vi "ITC503 -- scan ITC LTC state.vi"(6 "error logfile path":path, 7 "disable interaction with itc":T1(ring)=enum."do not use oxford ITC", 8 "error in":errorcluster, 11 "state IN":T3={"LTC21 Address"="GPIB0::15::INSTR", "ITC503 Address"="GPIB0::24::INSTR", "ITC temperature"=138.96, "ITC set temperature"=55.0, "LTC temperature"=137.354, "heater"=0.0, "gas flow"=96.8, "P"=10.0, "D"=1.0, "I"=3.0, "ITC state"="X0A1C2S01H1L0\r", "nonzero temperature"=0.0, "Magn Field (T)"=0.0, "LakeShore340"="", "LS340 Adress"=0, "Sample Temperature Source"=enum."read T <- LakeShore 340", "Neocera sensor"=1}) -> (0 "error out":errorcluster, 1 "itc box state OUT":T2={"ITC503 Address"="GPIB0::15::INSTR", "ITC temperature"=0.0, "ITC set temperature"=300.0, "heater"=300.0, "gas flow"=1.6, "P"=0.0, "D"=10.0, "I"=0.1, "ITC state"="X0A1C2S01H1L0\r", "nonzero temperature"=0.0, "Magn Field (T)"=0.0}, 3 "state OUT":T3={"LTC21 Address"="GPIB0::15::INSTR", "ITC503 Address"="GPIB0::24::INSTR", "ITC temperature"=138.96, "ITC set temperature"=55.0, "LTC temperature"=137.354, "heater"=0.0, "gas flow"=96.8, "P"=10.0, "D"=1.0, "I"=3.0, "ITC state"="X0A1C2S01H1L0\r", "nonzero temperature"=0.0, "Magn Field (T)"=0.0, "LakeShore340"="", "LS340 Adress"=0, "Sample Temperature Source"=enum."read T <- LakeShore 340", "Neocera sensor"=1})   [LabVIEW 2014]
uses:
  state.ctl
  Sample_Temperature_Source_Control.ctl
  itc 503 box state.ctl
  itc 503 box - control.ctl
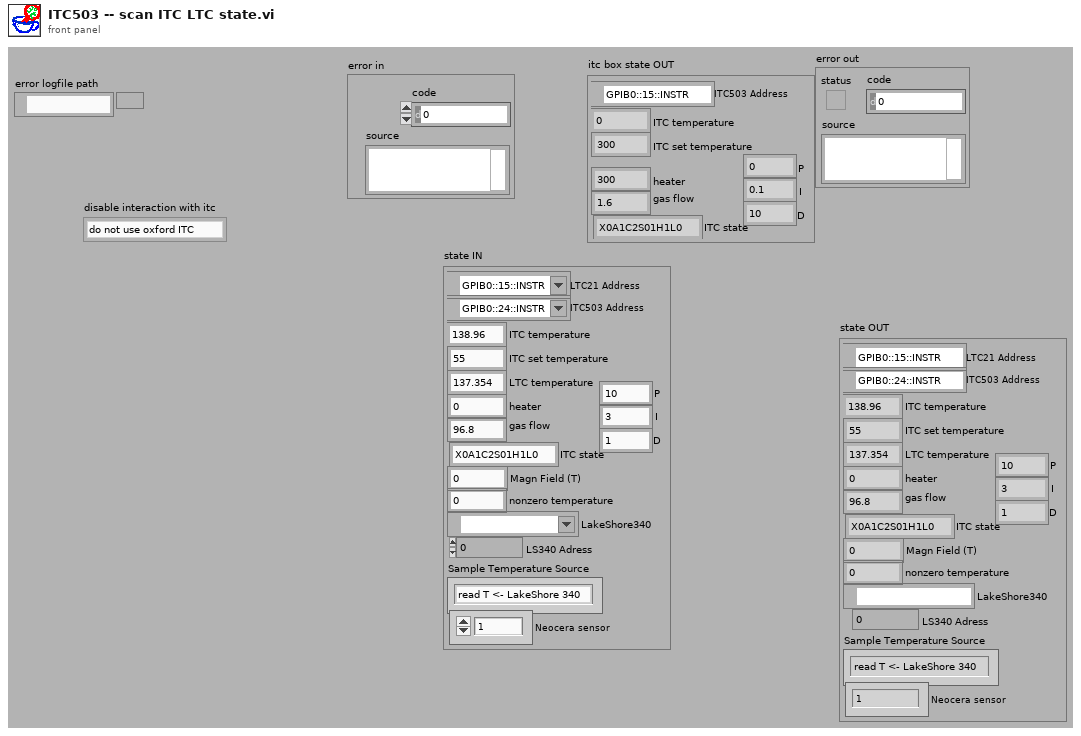
[diagram p1: front panel]
types:
  T1 = enum16{"use oxford ITC", "do not use oxford ITC"}
  T2 = typedef "itc 503 box state.ctl" = cluster{"ITC503 Address":refnum<visa-resource-name>, "ITC temperature":dbl, "ITC set temperature":dbl, "heater":dbl, "gas flow":dbl, "P":dbl, "D":dbl, "I":dbl, "ITC state":string, "nonzero temperature":dbl, "Magn Field (T)":dbl}
  T3 = typedef "state.ctl" = cluster{"LTC21 Address":refnum<visa-resource-name>, "ITC503 Address":refnum<visa-resource-name>, "ITC temperature":dbl, "ITC set temperature":dbl, "LTC temperature":dbl, "heater":dbl, "gas flow":dbl, "P":dbl, "D":dbl, "I":dbl, "ITC state":string, "nonzero temperature":dbl, "Magn Field (T)":dbl, "LakeShore340":refnum<visa-resource-name>, "LS340 Adress":i16, "Sample Temperature Source":T4, "Neocera sensor":i32}
  T4 = typedef "Sample_Temperature_Source_Control.ctl" = enum16{"read T <- LakeShore 340", "read T <- Neocera"}
  T5 = typedef "itc 503 box - control.ctl" = enum16{"heater manual and zero", "heater auto", "upload D", "upload I", "upload P", "shut off", "init", "read sweep table", "disable", "enable", "read state", "set gas to", "stop sweep", "start sweep", "test", "set temperature to", "write sweep table", "-void", "set heater to"}
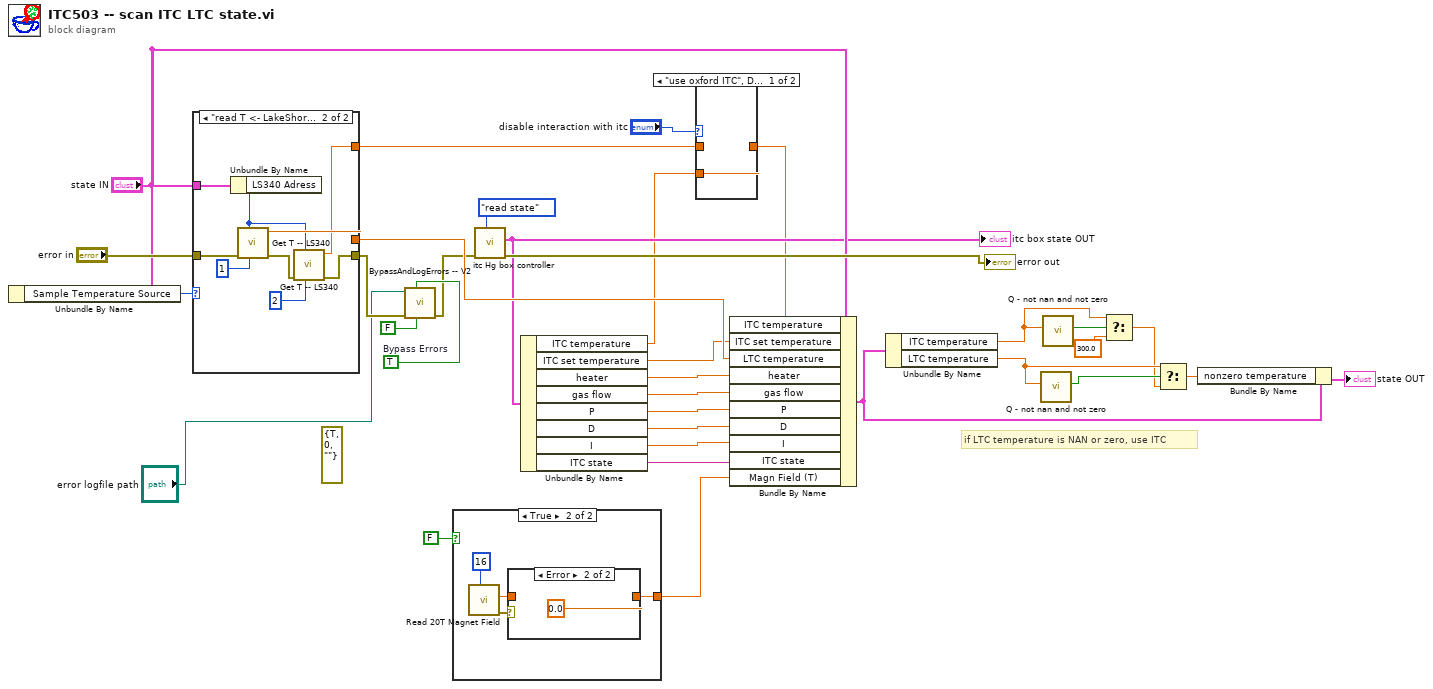
[diagram p0: block diagram]
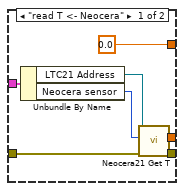
[diagram p3: hidden frame]
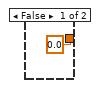
[diagram p4: hidden frame]
diagram:
  w5 = TRUE  # Bypass Errors
  (unwired) errorcluster {"status"=TRUE, "code"=0, "source"=""} ("error in")
  # "if LTC temperature is NAN or zero, use ITC"
  n1 = Unbundle By Name("state IN") -> ("Sample Temperature Source"=w13:T4)
  n2 = case shown="\"read T <- LakeShore 340\"" w13 {
    tunnel: [w41 w49] -> w34
    tunnel: "state IN" -> [w40 w50]
    tunnel: "error in" -> [w39 w48]
    tunnel: [w38 w44] -> w4
    tunnel: [0.0 w42] -> w8
    frame "read T <- Neocera" {
      n3 = Unbundle By Name(w40) -> ("LTC21 Address"=w37:refnum<visa-resource-name>, "Neocera sensor"=w36:i32)
      n4 = call "Neocera21 Get T.vi"("error in (no error)"=w39, "Sensor"=w36, "VISA Resource Name"=w37) -> ("error out"=w38:errorcluster, "Temperature"=w41:dbl)  [unwired: 5 in, 2 out]
    }
    frame "read T <- LakeShore 340" {
      n5 = Unbundle By Name(w50) -> ("LS340 Adress"=w43:i16)
      n6 = call "Get T -- LS340.vi"("sensor"=1, "GPIB Adress"=w43, "error in (no error)"=w48) -> ("error out"=w45:errorcluster, "sensor Temperature"=w49:dbl)  [unwired: 6 in, 1 out]
      n7 = call "Get T -- LS340.vi"("sensor"=2, "GPIB Adress"=w43, "error in (no error)"=w45) -> ("error out"=w44:errorcluster, "sensor Temperature"=w42:dbl)  [unwired: 6 in, 1 out]
    }
  }
  n8 = call "BypassAndLogErrors -- V2.vi"("Log Error ?"=FALSE, "Bypass Errors"=w5, "error in (no error)"=w4, "Log File Path"="error logfile path") -> ("error out"=w3:errorcluster)  [unwired: 7 in]
  n9 = case shown="True" FALSE {
    tunnel: [0.0 w52] -> w15
    frame False {
    }
    frame True {
      n10 = call "Read 20T Magnet Field.vi"("GPIB Adress"=i16 16) -> ("error out"=w54:errorcluster, "Magnetic Field (Tesla)"=w53:dbl)  [unwired: 8 in, 1 out]
      n11 = case shown="Error" w54 {
        tunnel: [w56 0.0] -> w52
        tunnel: w53 -> [w56 _]
        frame No Error {
        }
        frame Error {
        }
      }
    }
  }
  n12 = call "itc Hg box controller.vi"("itc box action"=itc_503_box_-_control."read state", "error in"=w3) -> ("error out"=→"error out":errorcluster, "itc box state OUT"=w10:T2)  [unwired: 7 in, 1 out]
  "itc box state OUT" <- w10
  n13 = Unbundle By Name(w10) -> ("ITC temperature"=w6:dbl, "ITC set temperature"=w22:dbl, "heater"=w21:dbl, "gas flow"=w20:dbl, "P"=w19:dbl, "D"=w18:dbl, "I"=w17:dbl, "ITC state"=w16:string)
  n14 = case shown="\"use oxford ITC\", Default" "disable interaction with itc" {
    tunnel: w8 -> [_ w59]
    tunnel: [w58 w59] -> w7
    tunnel: w6 -> [w58 _]
    frame "use oxford ITC", Default {
    }
    frame "do not use oxford ITC" {
    }
  }
  n15 = Bundle By Name(cluster="state IN", "ITC temperature"=w7, "ITC set temperature"=w22, "LTC temperature"=w34, "heater"=w21, "gas flow"=w20, "P"=w19, "D"=w18, "I"=w17, "ITC state"=w16, "Magn Field (T)"=w15) -> (w32:T3)
  n16 = Unbundle By Name(w32) -> ("ITC temperature"=w27:dbl, "LTC temperature"=w29:dbl)
  n17 = call "Q - not nan and not zero.vi"("Numeric"=w29) -> ("Boolean"=w30:bool)  [unwired: 10 in]
  n18 = call "Q - not nan and not zero.vi"("Numeric"=w27) -> ("Boolean"=w28:bool)  [unwired: 10 in]
  n19 = Select(t=w27, s=w28, f=300.0) -> (s? t:f=w25:dbl)
  n20 = Select(t=w29, s=w30, f=w25) -> (s? t:f=w24:dbl)
  n21 = Bundle By Name(cluster=w32, "nonzero temperature"=w24) -> (→"state OUT":T3)
